vi "Internal_triggers_logic.vi"(5 "Imaging Protocol":T1=enum."Live Imaging", 6 "aol_ref_scan_next":bool, 7 "Trigger 1 selector":T2, 8 "Start":bool, 9 "Line_signal":bool, 10 "End of trial":bool, 11 "Repeat trigger":bool) -> (0 "Trigger In":bool, 1 "Trigger pulse (pos. edge)":bool, 2 "Trial start trigger signal":bool, 3 "Encoder trigger signal":bool)   [LabVIEW 2020]
uses:
  Typedefs/Trigger 1 selector enum.ctl
  Typedefs/Imaging Protocols enum.ctl
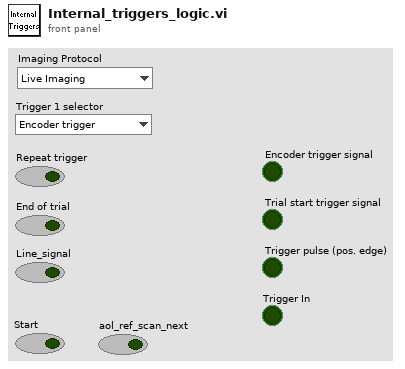
[diagram p1: front panel]
types:
  T1 = typedef "Imaging Protocols enum.ctl" = enum16{"AOL Z-Stack", "Motor Z Stack", "Functional Acquisition", "Single Plane Acquisition", "Volume Acquisition", "Live Imaging", "Live Plane Imaging", "Live Volume Imaging"}
  T2 = typedef "Trigger 1 selector enum.ctl" = enum16{"Encoder trigger", "Line trigger", "Control system's ref frame acknowledgement"}
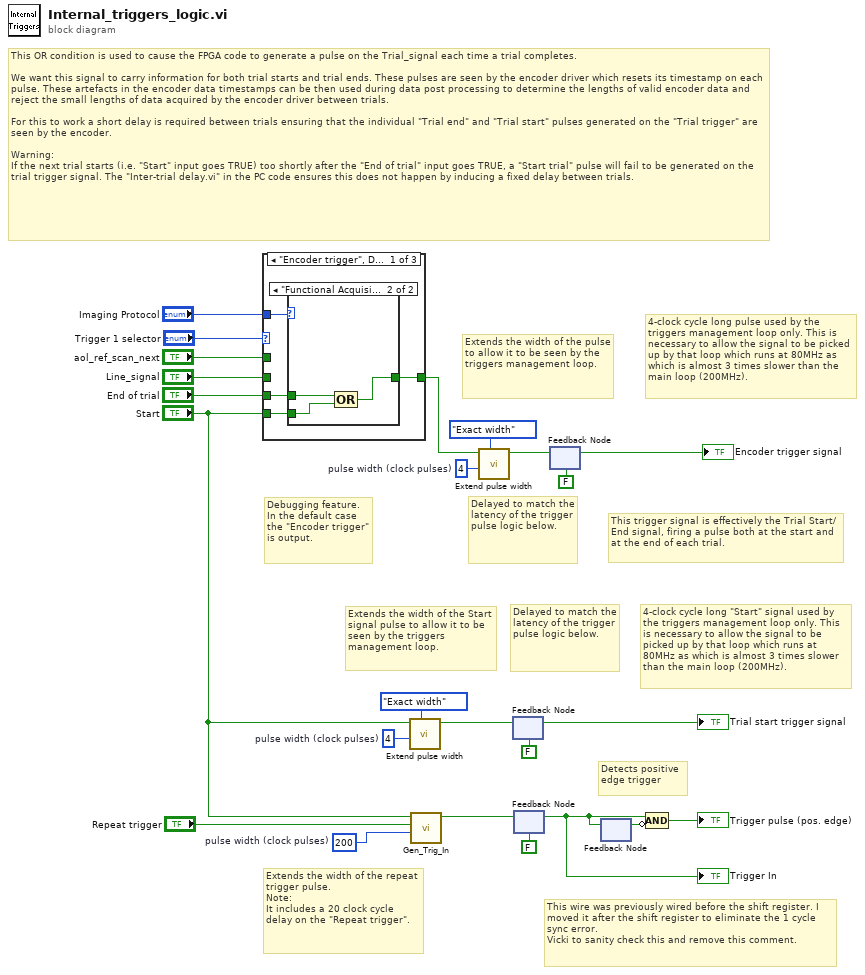
[diagram p0: block diagram]
diagram:
  w12 = u32 4  # pulse width (clock pulses)
  w17 = u32 4  # pulse width (clock pulses)
  w22 = u8 200  # pulse width (clock pulses)
  # "Debugging feature.\nIn the default case the \"Encoder trigger\" is output."
  # "This trigger signal is effectively the Trial Start/End signal, firing a pulse both at the start and at the end of each trial."
  # "Delayed to match the latency of the trigger pulse logic below."
  # "4-clock cycle long pulse used by the triggers management loop only. This is necessary to allow the signal to be picked up by that loop which runs at 80MHz as which is almost 3 times slower than the main loop (200MHz)."
  # "Extends the width of the pulse to allow it to be seen by the triggers management loop."
  # "This OR condition is used to cause the FPGA code to generate a pulse on the Trial_signal each time a trial completes.\n\nWe want this signal to carry information for both trial starts and trial ends. These pulses are seen by the encoder driver which resets its timestamp on each pulse. These artefacts in the encoder data timestamps can be then used during data post processing to determine the lengths of valid encoder data and reject the small lengths of data acquired by the encoder driver between trials.\n\nFor this to work a short delay is required between trials ensuring that the individual \"Trial end\" and \"Trial start\" pulses generated on the \"Trial trigger\" are seen by the encoder.\n\nWarning:\nIf the next trial starts (i.e. \"Start\" input goes TRUE) too shortly after the \"End of trial\" input goes TRUE, a \"Start trial\" pulse will fail to be generated on the trial trigger signal. The \"Inter-trial delay.vi\" in the PC code ensures this does not happen by inducing a fixed delay between trials."
  # "This wire was previously wired before the shift register. I moved it after the shift register to eliminate the 1 cycle sync error.\nVicki to sanity check this and remove this comment."
  # "Delayed to match the latency of the trigger pulse logic below."
  # "4-clock cycle long \"Start\" signal used by the triggers management loop only. This is necessary to allow the signal to be picked up by that loop which runs at 80MHz as which is almost 3 times slower than the main loop (200MHz)."
  # "Extends the width of the Start signal pulse to allow it to be seen by the triggers management loop."
  # "Extends the width of the repeat trigger pulse.\nNote:\nIt includes a 20 clock cycle delay on the \"Repeat trigger\"."
  # "Detects positive edge trigger"
  n1 = case shown="\"Encoder trigger\", Default" "Trigger 1 selector" {
    tunnel: [w27 w33 w34] -> w6
    tunnel: "Line_signal" -> [_ w33 _]
    tunnel: "aol_ref_scan_next" -> [_ _ w34]
    tunnel: "Imaging Protocol" -> [w28 _ _]
    tunnel: "Start" -> [w26 _ _]
    tunnel: "End of trial" -> [w25 _ _]
    frame "Encoder trigger", Default {
      n2 = case shown="\"Functional Acquisition\"" w28 {
        tunnel: [w29 w32] -> w27
        tunnel: w26 -> [w29 w31]
        tunnel: w25 -> [_ w30]
        frame Default {
          # "Handles live imaging encoder triggering."
        }
        frame "Functional Acquisition" {
          n3 = Compound Arithmetic op=OR(w30, w31) -> (w32:bool)
        }
      }
    }
    frame "Line trigger" {
    }
    frame "Control system's ref frame acknowledgement" {
    }
  }
  n4 = call "Extend pulse width.vi"("Function"=enum16{"Minimum width", "Exact width"}."Exact width", "Pulse width (ticks)(80000=1ms @80MHz)"=w17, "Input signal"="Start") -> ("Output signal"=w19:bool)  [unwired: 8 in]
  n5 = call "Gen_Trig_In.vi"("Pulse width (clock pulses)"=w22, "Repeat Trigger"="Repeat trigger", "Start"="Start") -> ("Output"=w16:bool)  [unwired: 8 in]
  n6 = call "Extend pulse width.vi"("Function"=enum16{"Minimum width", "Exact width"}."Exact width", "Pulse width (ticks)(80000=1ms @80MHz)"=w12, "Input signal"=w6) -> ("Output signal"=w10:bool)  [unwired: 8 in]
  n7 = feedback #1(FALSE) -> (→"Trial start trigger signal":bool)
  n8 = feedback-in #1(w19) -> ()
  n9 = feedback #2(FALSE) -> (w13:bool)
  "Trigger In" <- w13
  n10 = feedback-in #2(w16) -> ()
  n11 = feedback #3(FALSE) -> (→"Encoder trigger signal":bool)
  n12 = feedback-in #3(w10) -> ()
  n13 = feedback #4() -> (w15:bool)  [unwired: 1 in]
  n14 = feedback-in #4(w13) -> ()
  n15 = Compound Arithmetic op=AND(w13, invert w15) -> (→"Trigger pulse (pos. edge)":bool)
